vi "Get Child IDs.vi"(7 "Linked List ID":string, 8 "error in (no error)":errorcluster, 11 "Linked List in":refnum<class "Linked List.lvclass">) -> (0 "error out":errorcluster, 2 "Child IDs":string[](array[string]), 3 "Linked List out":refnum<class "Linked List.lvclass">)   [LabVIEW 2019, in "Linked Lists.lvlib" / "Linked List.lvclass"]
uses:
  <vilib>/gpm_packages/@cs/linked-list/Source/Linked List/Linked List/Linked List.lvclass
  <vilib>/gpm_packages/@cs/linked-list/Source/Linked List/Linked List Definition/Linked List Definition.lvclass
  <vilib>/gpm_packages/@cs/linked-list/Source/Linked List/Linked List/Linked List.lvclass/Linked List.ctl
  <vilib>/gpm_packages/@cs/lookup-table/Source/LookupTable/LookupTable.lvclass/LookupTable.ctl
  3d7f4a9a-e650-4d06-8acf-6c8a7b50f671.vi
  <vilib>/gpm_packages/@cs/lookup-table/Source/LookupTable/Read Table Reference.vi
  3d7f4a9a-e650-4d06-8acf-6c8a7b50f671.vi/8ec13971-d60f-4a19-ad63-966c04ae4816.vi
  <vilib>/gpm_packages/@cs/lookup-table/Source/LookupTable/LookupTable.lvclass
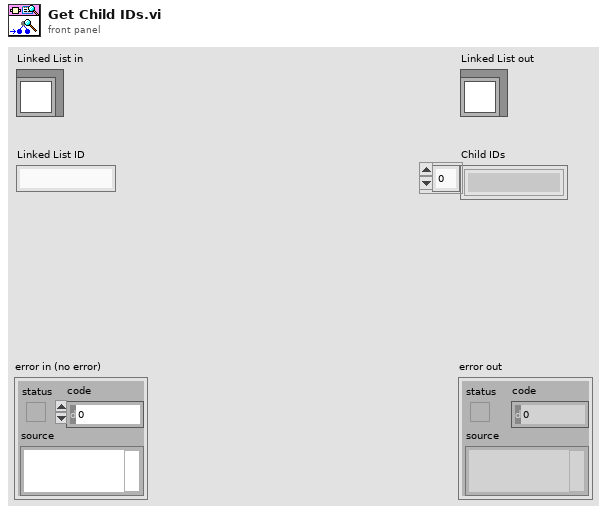
[diagram p1: front panel]
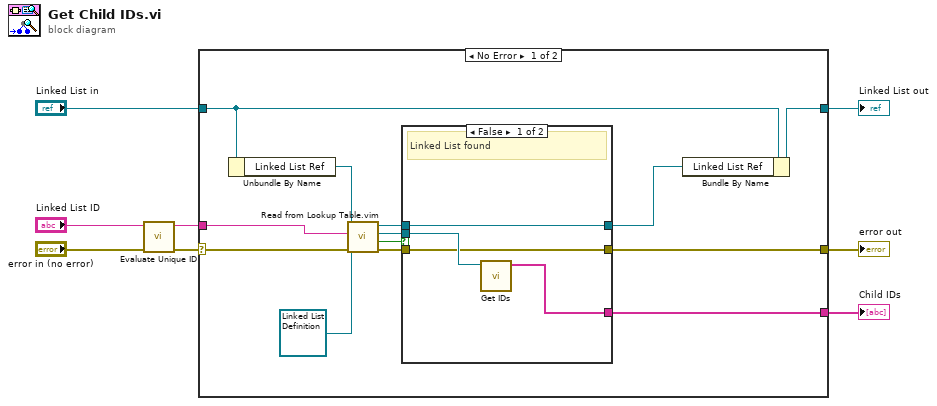
[diagram p0: block diagram]
diagram:
  n1 = call <vilib>:"Evaluate Unique ID.vi"("error in (no error)"="error in (no error)", "Unique ID"="Linked List ID") -> ("error out"=w6:errorcluster, "Unique ID Out"=w5:string)  [unwired: 8 in]
  n2 = case shown="No Error" w6 {
    selector: w6 -> [w21 w29]
    tunnel: w5 -> [w19 _]
    tunnel: "Linked List in" -> [w14 w28]
    tunnel: [w13 w28] -> w3
    tunnel: [w11 w29] -> w2
    tunnel: [w10 _] -> w1
    frame No Error {
      n3 = Unbundle By Name(w14) -> ("Linked List Ref"=w20:refnum<data-value>)
      n4 = call "Read from Lookup Table.vim"("error in (no error)"=w21, "Type"=refnum<class "Linked List Definition.lvclass"> refnum ("Linked List.lvlib:Linked List Definition.lvclass"), "Item Name"=w19, "LookupTable Reference"=w20) -> ("error out"=w18:errorcluster, "Not Found?"=w9:bool, "Value"=w15:refnum<class "Linked List Definition.lvclass">, "LookupTable Reference Out"=w17:refnum<data-value>)  [unwired: 4 in]
      n5 = case shown="False" w9 {
        tunnel: w18 -> [w23 w26]
        tunnel: w17 -> [w24 w27]
        tunnel: w15 -> [w25 _]
        tunnel: [w24 w27] -> w12
        tunnel: [w23 w26] -> w11
        tunnel: [w22 _] -> w10
        frame False {
          # "Linked List found"
          n6 = call <vilib>:"Get IDs.vi"("Linked List Definition in"=w25) -> ("Child IDs"=w22:string[])  [unwired: 8 in, 2 out]
        }
        frame True {
          # "Linked List not found"
        }
      }
      n7 = Bundle By Name(cluster=w14, "Linked List Ref"=w12) -> (w13:refnum<class "Linked List.lvclass">)
    }
    frame Error {
    }
  }
  "error out" <- w2
  "Linked List out" <- w3
  "Child IDs" <- w1
